vi "Send Initiate Generation.vi"(7 "Message Priority (Normal)":T1=enum."Normal", 8 "error in (no error)":errorcluster, 10 "Execute?":bool, 11 "Message Enqueuer":refnum<class "Message Enqueuer.lvclass">) -> (0 "error out":errorcluster, 3 "Message Enqueuer out":refnum<class "Message Enqueuer.lvclass">)   [LabVIEW 2015, in "CS++Fgen.lvlib" / "Initiate Generation Msg.lvclass"]
doc: "Sends the <B>CS++Fgen.lvlib:Initiate Generation Msg.lvclass</B> message.\n\n<B>CS++Fgen.lvlib:CS++Fgen.lvclass:Initiate Generation.vi</B> Description:\n\nThis VI initiates signal generation. If the function generator is in the Configuration State, this VI moves the function generator to the Output Generation State. If the function generator is already in the Output Generation State, this VI does nothing.\n\nThe instrument is in the Generation State after you call the IviFgen Initialize, IviFgen Initialize With Options, or IviFgen Reset VIs. You can configure the output of the function generator regardless of whether function generator is in the Configuration State or the Generation State. This means that you are required to call the IviFgen Initiate Generation VI only if you abort signal generation by calling the IviFgen Abort Generation VI. \n\nMany function generators constantly generate an output signal, and do not require you to initiate signal generation. If a function generator is always outputting the currently configured signal, this VI does nothing.\n\nYou are not required to call the IviFgen Initiate Generation and IviFgen Abort Generation VIs. Whether you choose to call these VIs in an application program has no impact on interchangeability. You can choose to use these VIs if you want to optimize your application for instruments that exhibit increased performance when output configuration is performed while the instrument is not generating a signal.\n\nThis VI disables extensions that have not been set by the user under the following conditions:\n\n(1) If you have not set the value of any property in the IviFgenModulateAM extension on a channel, this VI sets the IviFgen>>Amplitude Modulation Attributes>>AM Enabled [AM] property to FALSE for that channel.\n\n(2) If you have not set the value of any property in the IviFgenModulateFM extension on a channel, this VI sets the IviFgen>>Frequency Modulation Attributes>>FM Enabled [FM] property to FALSE for that channel.\n\nNotes:\n\n(1) This VI does not normally check the instrument status. Typically, you call this VI only in a sequence of calls to other low-level driver functions. The sequence performs one operation. You use the low-level VIs to optimize one or more aspects of interaction with the instrument. If you want to check the instrument status, call the IviFgen Error-Query VI at the conclusion of the sequence.\n\n(2) This VI performs interchangeability checking when the IviFgen>>Inherent IVI Settings>>User Options>>Interchange Check property is set to TRUE. If the IviFgen>>Inherent IVI Settings>>User Options>>Spy property is set to TRUE, you use the NI I/O Trace utility to view interchangeability warnings. You use the IviFgen Get Next Interchange Warning VI to retrieve interchangeability warnings when the IviFgen>>Inherent IVI Settings>>User Options>>Spy property is set to FALSE. For more information about interchangeability checking, refer to the help text for the IviFgen>>Inherent IVI Settings>>User Options>>Interchange Check property."
uses:
  Initiate Generation Msg.lvclass
  <vilib>/ActorFramework/Message Enqueuer/Message Enqueuer.lvclass
  <vilib>/ActorFramework/Message Enqueuer/Message Priority.ctl
  Initiate Generation Msg.lvclass/Initiate Generation Msg.ctl
  <vilib>/ActorFramework/Message Enqueuer/Message Enqueuer.lvclass/Message Enqueuer.ctl
  <vilib>/ActorFramework/Message Priority Queue/Priority Enqueue.vi
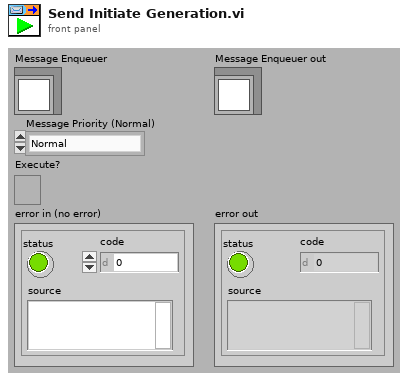
[diagram p1: front panel]
types:
  T1 = typedef "Actor Framework.lvlib/Message Enqueuer.lvclass/Message Priority.ctl" = enum16{"Low", "Normal", "High"}
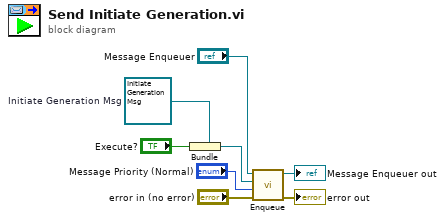
[diagram p0: block diagram]
diagram:
  w2 = refnum<class "Initiate Generation Msg.lvclass"> refnum  # Initiate Generation Msg
  n1 = Bundle(cluster=w2, "Execute?") -> (w5:refnum<class "Initiate Generation Msg.lvclass">)
  n2 = call <vilib>:"Enqueue.vi"("error in (no error)"="error in (no error)", "Message Priority (Normal)"="Message Priority (Normal)", "Message"=w5, "Message Enqueuer in"="Message Enqueuer") -> ("error out"=→"error out":errorcluster, "Message Enqueuer out"=→"Message Enqueuer out":refnum<class "Message Enqueuer.lvclass">)  [unwired: 6 in]
